vi "FA25_FW_pendulum_L3_4_0.vi"() -> ()   [LabVIEW 2024]
uses:
  <vilib>/Analysis/3filter.llb/Filter Passband Type.ctl
  SADI_Pendulum_lib/pendulumApp.lvlib
  <vilib>/ptbypt/NI_PtbyPt.lvlib
  <vilib>/Analysis/NI_AALBase.lvlib
panel:
  in  "Tab Control":T1(tab)=enum."Plant and Controller"
  out "Firmware Version":sgl=1.002
  out "Software Version":dbl=1.104 format="%_6g"
  out "Number of SADI":i32=1
  out "reset":i32
  out "SADI Connect":i32
  out "P query":i32
  out "P start":i32
  in  "Desired DAQ Loop \nTime (ms)":dbl=0.2
  out "Actual DAQ Loop \nTime (ms)":dbl=0.20860000000084256 format="%#_7g"
  out "Elapsed \nTime (s) daq loop":dbl=15.046546899999953
  out "Txlat_ms":dbl=1.778
  out "min Txlat":dbl=0.682 format="%0.6f"
  out "max TXlat":dbl=4.932 format="%0.6f"
  out "std dev TXlat":dbl=0.7050052541669608 format="%0.6f"
  out "mean  TXlat":dbl=1.2022235999999924 format="%0.6f"
  out "Tx latency, ms":T2(graph)={"X Values"=[0.70325, 0.74575, 0.7882500000000001, 0.8307500000000001, 0.8732500000000001, 0.9157500000000001, 0.95825, 1.00075, 1.04325, 1.0857500000000002, 1.1282500000000002, 1.1707500000000002, 1.2132500000000002, 1.2557500000000001, 1.2982500000000001, 1.34075, 1.38325, 1.42575, 1.46825, 1.51075, 1.55325, 1.59575, 1.63825, 1.68075, 1.72325, 1.76575, 1.8082500000000004, 1.8507500000000003, 1.8932500000000003, 1.9357500000000003, 1.9782500000000003, 2.02075, 2.06325, 2.10575, 2.14825, 2.19075, 2.23325, 2.27575, 2.31825, 2.36075, 2.40325, 2.44575, 2.48825, 2.53075, 2.57325, 2.61575, 2.65825, 2.7007499999999998, 2.7432499999999997, 2.7857499999999997, 2.8282499999999997, 2.8707499999999997, 2.9132499999999997, 2.95575, 2.99825, 3.04075, 3.08325, 3.12575, 3.16825, 3.21075, 3.25325, 3.29575, 3.33825, 3.38075, 3.42325, 3.46575, 3.50825, 3.55075, 3.59325, 3.63575, 3.67825, 3.72075, 3.7632499999999998, 3.8057499999999997, 3.84825, 3.89075, 3.93325, 3.97575, 4.01825, 4.0607500000000005, 4.10325, 4.1457500000000005, 4.18825, 4.2307500000000005, 4.27325, 4.31575, 4.35825, 4.40075, 4.44325, 4.48575, 4.52825, 4.57075, 4.61325, 4.65575, 4.698250000000001, 4.74075, 4.783250000000001, 4.82575, 4.868250000000001, 4.91075], "Histogram: h(x)"=[155, 338, 552, 840, 858, 795, 153, 0, 0, 0, 0, 0, 0, 0, 0, 0, 0, 0, 0, 0, 0, 0, 0, 5, 49, 156, 220, 199, 196, 149, 0, 0, 0, 0, 0, 0, 0, 0, 0, 0, 0, 0, 0, 0, 0, 0, 0, 17, 26, 34, 37, 44, 58, 6, 0, 0, 0, 0, 0, 0, 0, 0, 0, 0, 0, 0, 0, 0, 0, 0, 0, 5, 5, 19, 5, 41, 7, 0, 0, 0, 0, 0, 0, 0, 0, 0, 0, 0, 0, 0, 0, 0, 0, 0, 0, 4, 0, 3, 0, 24]}
  out "ENC VEL":dbl=0.5175486320891765
  out "Pend Rot Error":dbl
  out "Pend Rot Filt":dbl=nan format="%0.2f"
  out "Pendulum velocity":dbl=3.5305560095629e-285
  out "Platen velocity":dbl=0.01738392532814515
  out "Command":dbl=-14.479572053947942
  out "desired\nposition":dbl=-14.790379679306856
  out "Platen Rot Error":dbl format="%0.2f"
  in  "Frequency":dbl=0.5
  in  "Amplitude":dbl=100.0
  in  "Turn On Command":dbl=40.0
  in  "Stop":bool=TRUE
  in  "Desired Loop \nTime (ms)":dbl=1.0
  out "Actual Loop Time (ms)":dbl=1.0000979999995252
  out "Elapsed Time (s)":dbl=15.048252700000035
  out "Segments Saved":u32
  in  "Save Data?":bool
  out "ENC POS":i32=-761
  out "Pendulum ENC":i32
  in  "Sine/Square":bool=TRUE
  in  "Enable Motor":bool=TRUE
  in  "Output Units":enum16{"Degrees", "Radians"}(ring)
  in  "Couts/rev":dbl=3704.0
  in  "Zero":bool
  out "Platen Rotation":dbl=-73.96328293736501
  out "Command Graph":T3(graph)={"Desired Rotation/Command"=-14.479572053947942, -14.479572053947942, 0.0, 0.0}
  out "Desired vs Actual Platen Angle Graph":cluster{"sine wave":dbl, "Filtered x":dbl}(graph)={"sine wave"=-14.479572053947942, "Filtered x"=-73.96328293736501}
  out "Pendulum Rotation Graph":cluster{dbl, dbl}(graph)={nan, 0.0}
  in  "n-int":i32=100
  in  "n-diff":i32=5
  in  "Sampling freq: fs":dbl=1000.0
  in  "Cutoff freq: fl":dbl=10.0 format="%0.3f"
  in  "initialize":bool
  out "PendEncValMax":u16=3687
  out "PendEncValMin":u16=3178
  in  "Pendulum Zero":bool
  out "Pend Rotation":dbl=1440.0 format="%0.2f"
  out "Read Call Error Out":u16(ring)=32768 items=["SADI_RESET (FT_OK)"=0, "FT_INVALID_HANDLE"=1, "FT_DEVICE_NOT_FOUND"=2, "FT_DEVICE_NOT_OPENED"=3, "FT_IO_ERROR"=4, "FT_INSUFFICIENT_RESOURCES"=5, "FT_OTHER_ERROR"=18, "FT_NOT_SUPPORTED"=17, "DATA_RECEIVED"=32768, "NO_DATA_AVAIL"=32769, "NO_SADI"=32770]
  out "SADI State":T4(ring)=enum."Close"
  # "Platen Rotation & Velocity"
  # "Signal Generator"
  # "Butterworth Filter Settings"
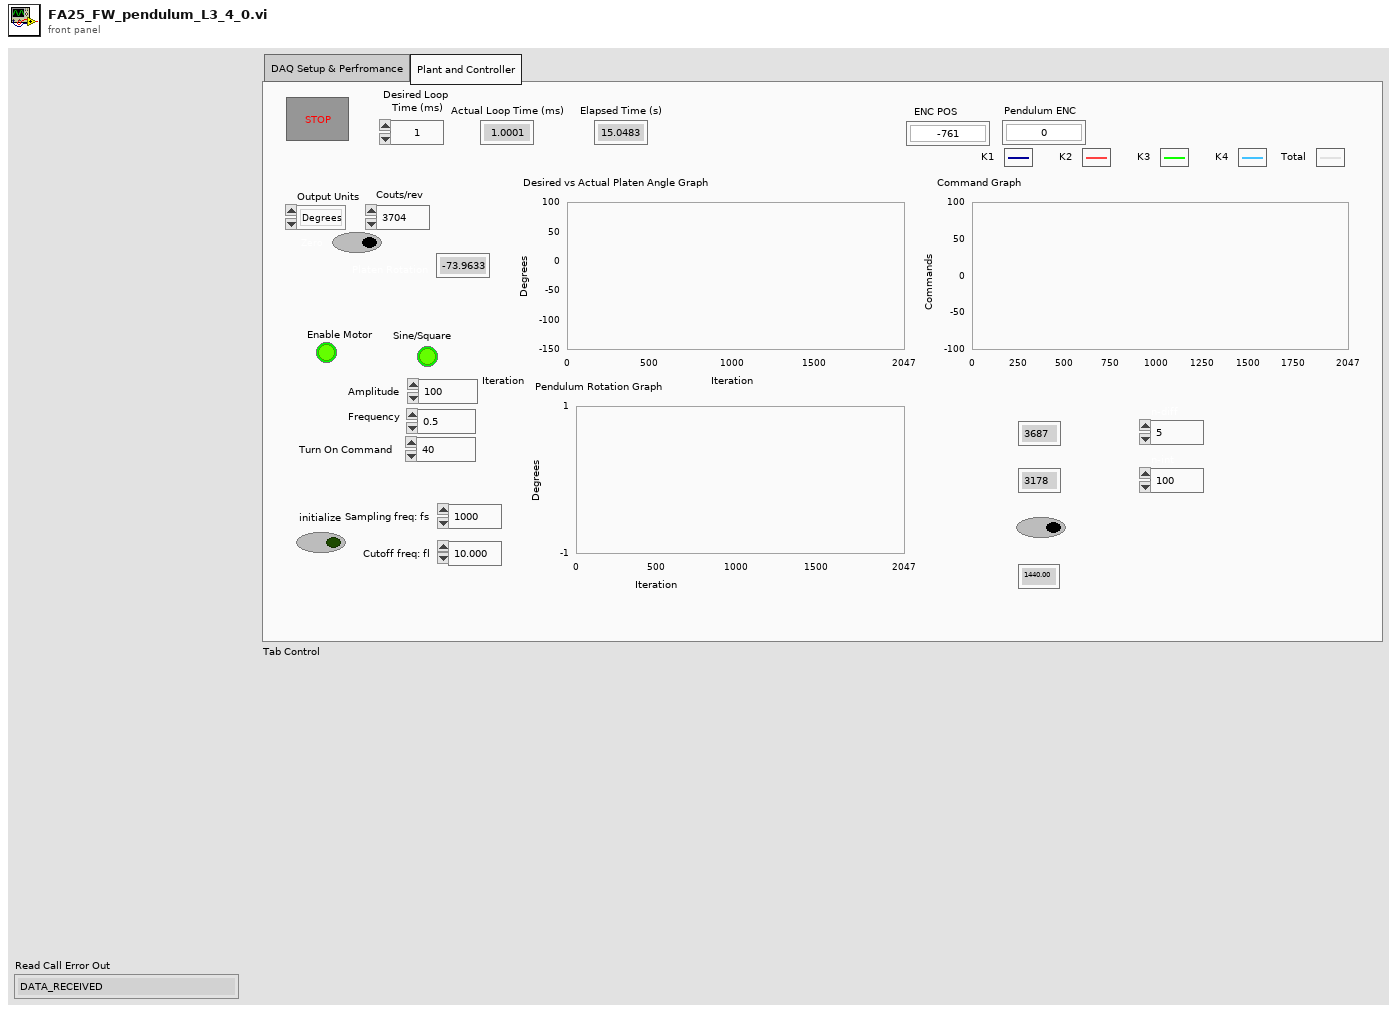
[diagram p1: front panel]
types:
  T1 = enum32{"DAQ Setup & Perfromance", "Plant and Controller"}
  T2 = cluster{"X Values":dbl[], "Histogram: h(x)":i32[]}
  T3 = cluster{"Desired Rotation/Command":dbl, dbl, dbl, dbl}
  T4 = enum32{"SADI_check", "Connect_boot", "Check_SW_FW", "Pend_Start", "Run", "Stop", "Store", "Close"}
  T5 = typedef "NI_AALBase.lvlib/Filter Passband Type.ctl" = enum32{"Lowpass", "Highpass", "Bandpass", "Bandstop"}
  T6 = cluster{"desired\nposition":dbl, "Platen Rotation":dbl}
  T7 = cluster{"desired\nposition":dbl, "Command":dbl, dbl, dbl}
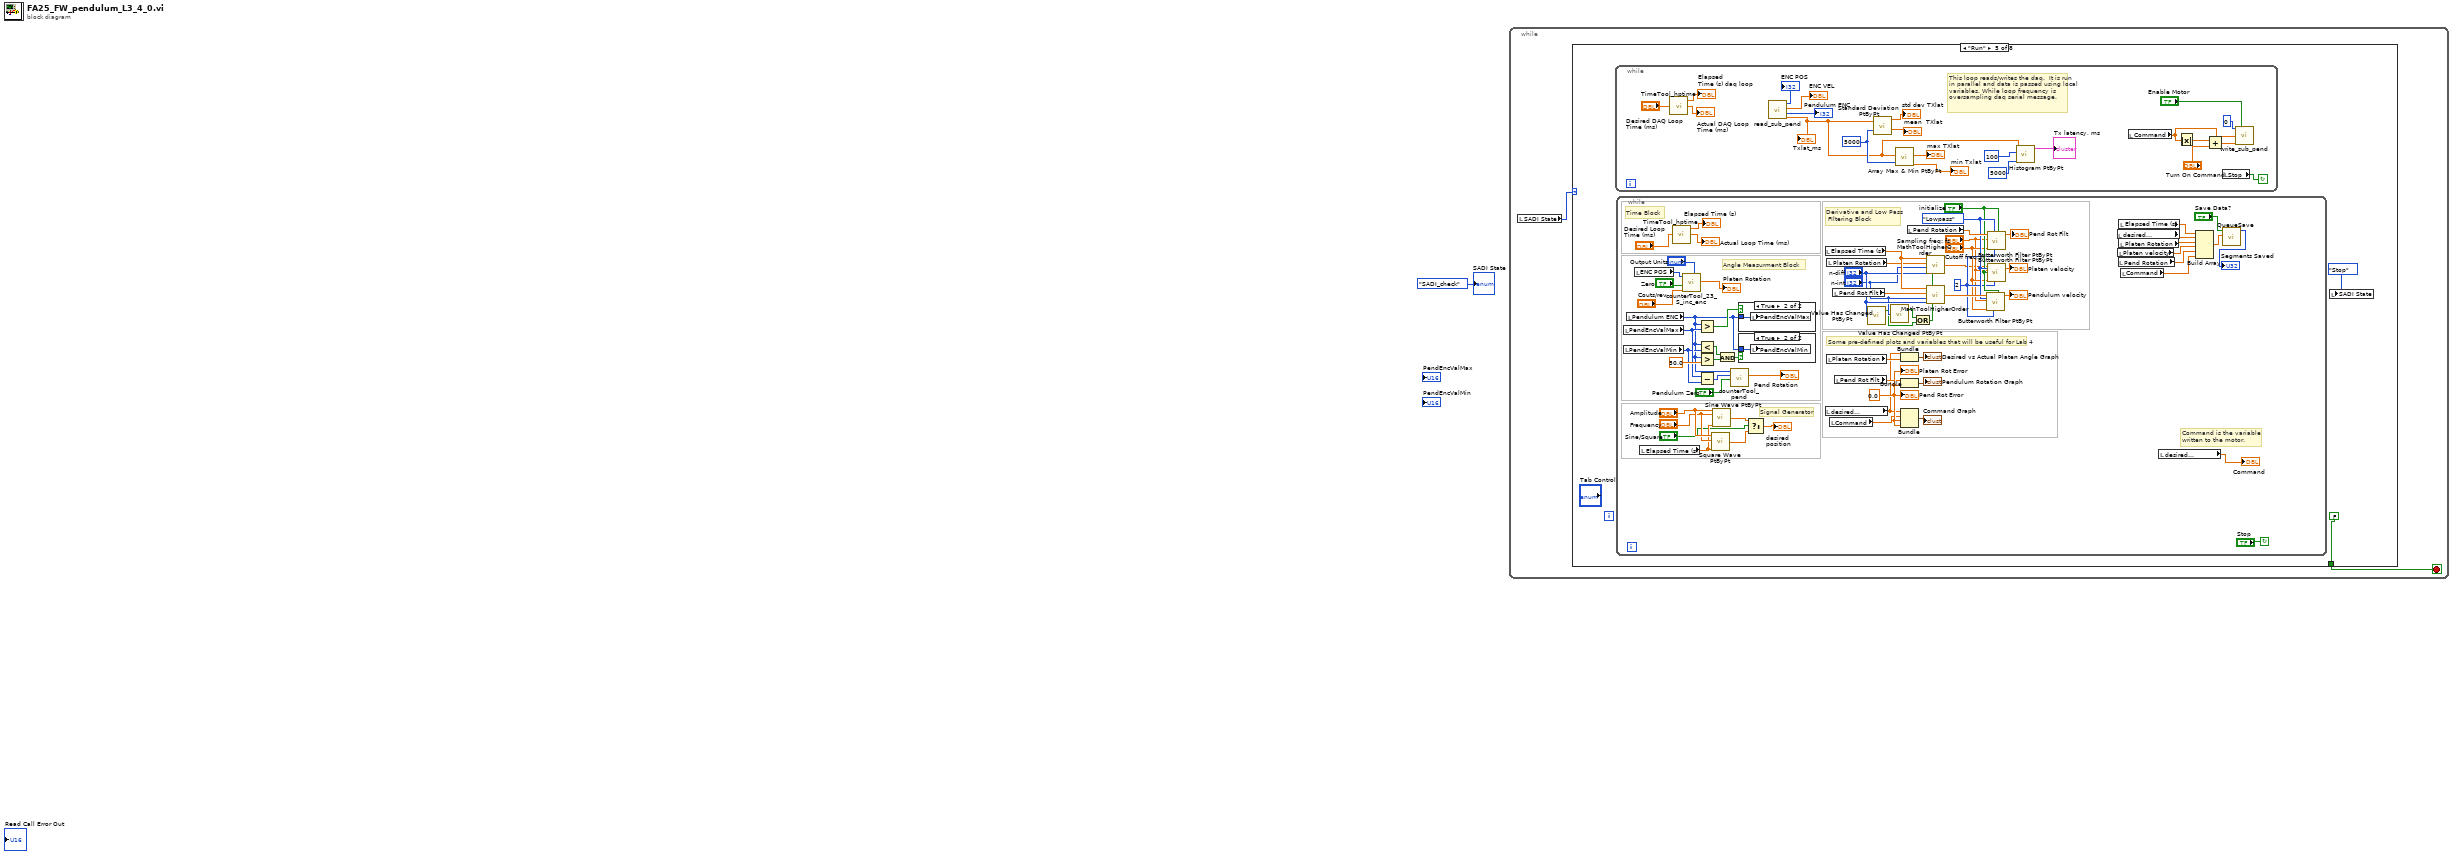
[diagram p0: block diagram]
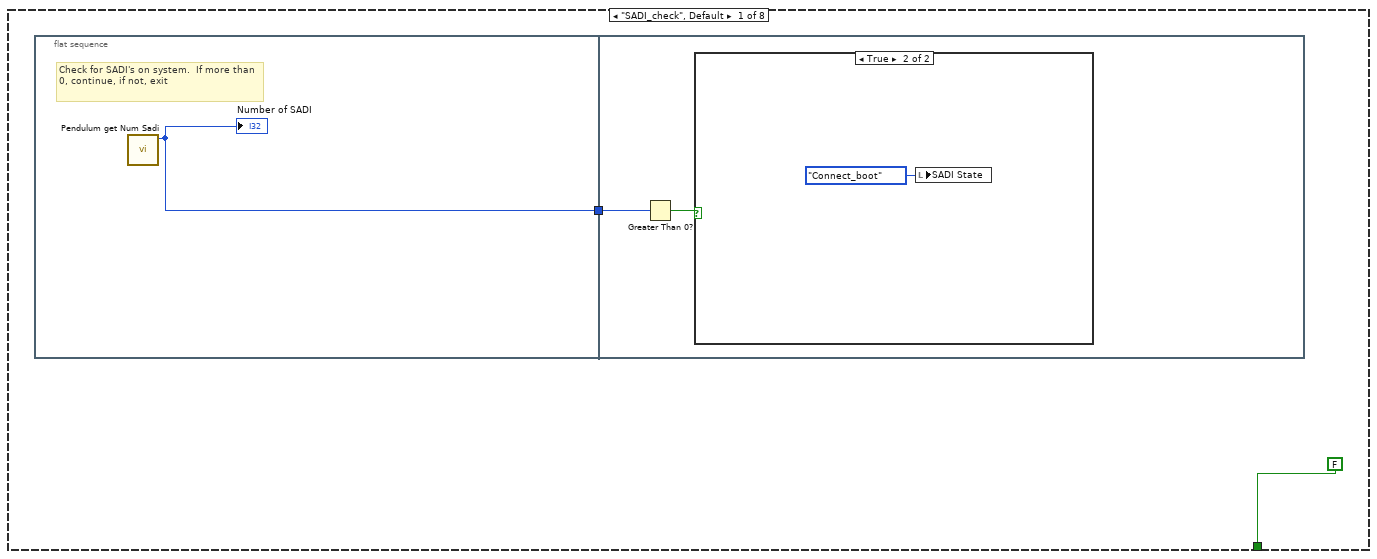
[diagram p2: hidden frame]
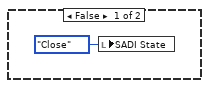
[diagram p3: hidden frame]
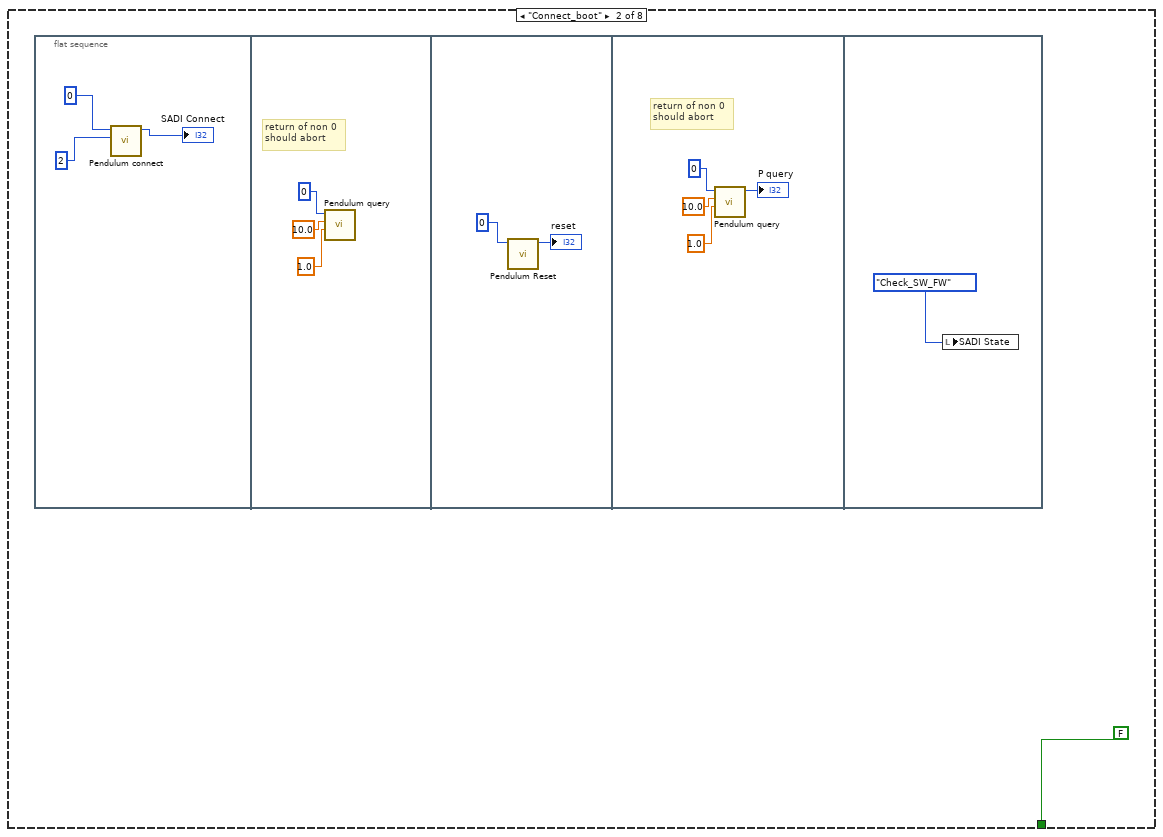
[diagram p4: hidden frame]
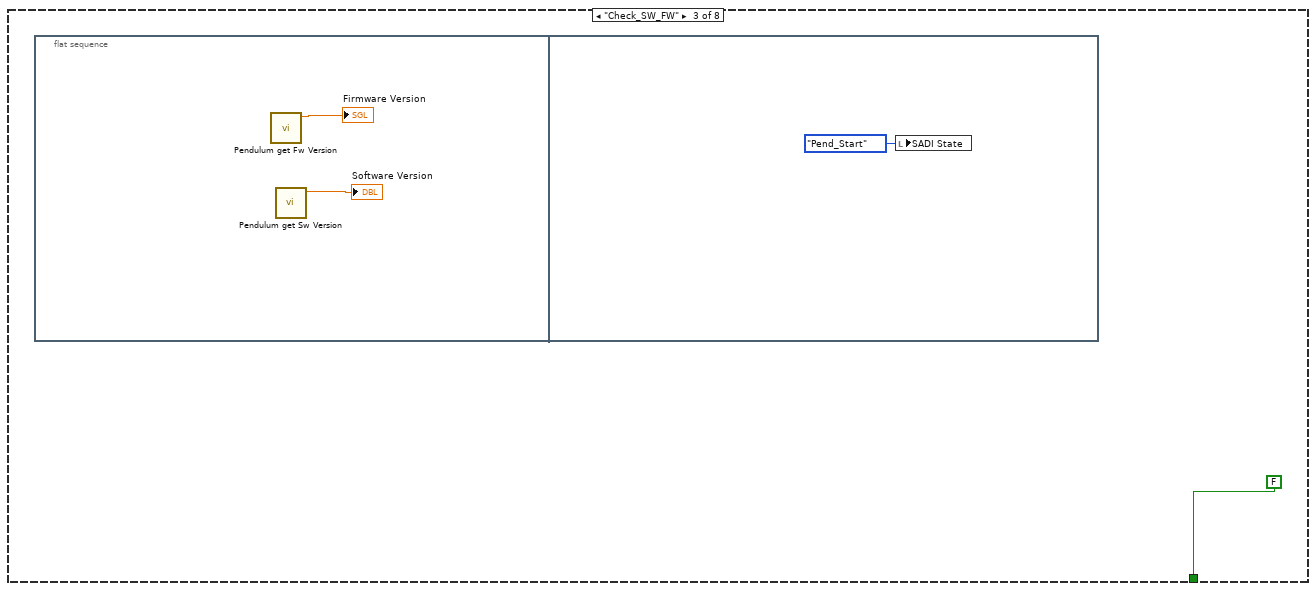
[diagram p5: hidden frame]
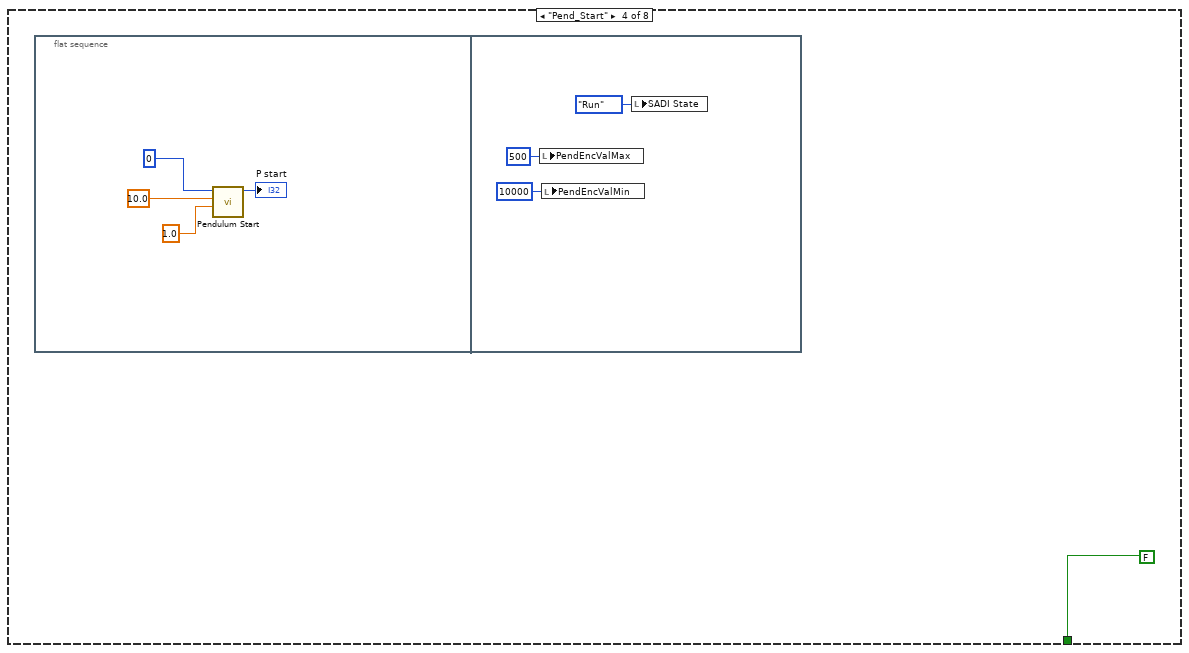
[diagram p6: hidden frame]
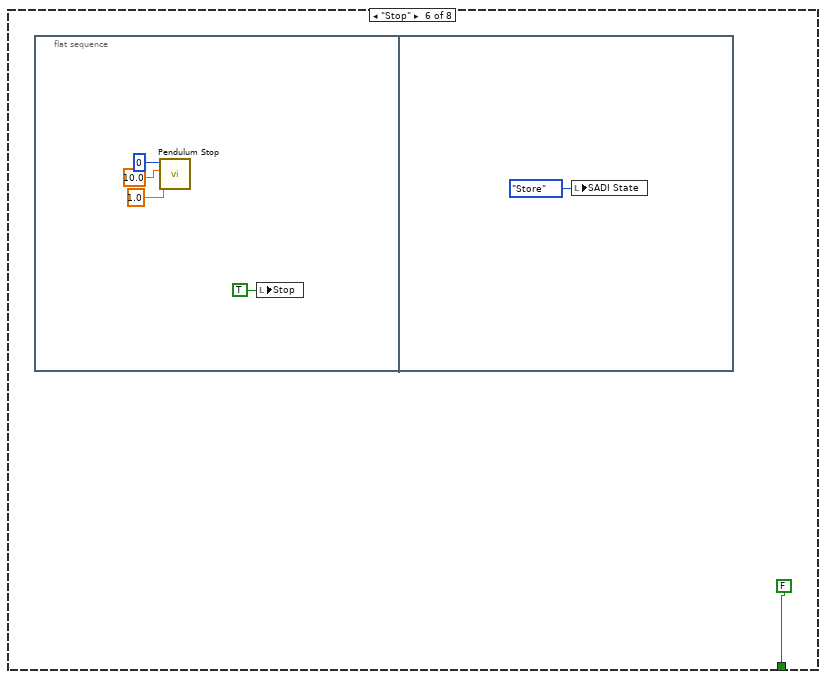
[diagram p9: hidden frame]
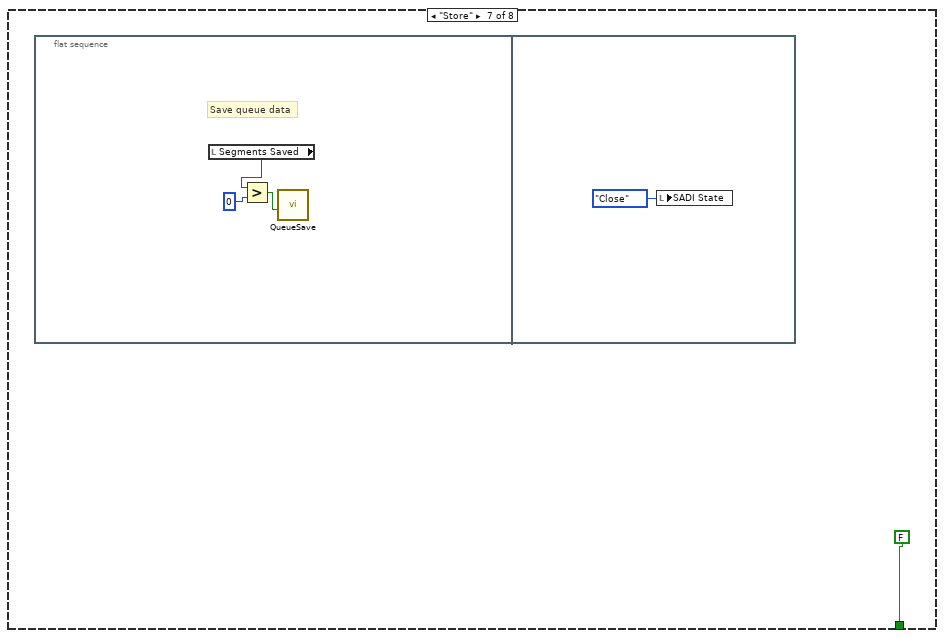
[diagram p10: hidden frame]
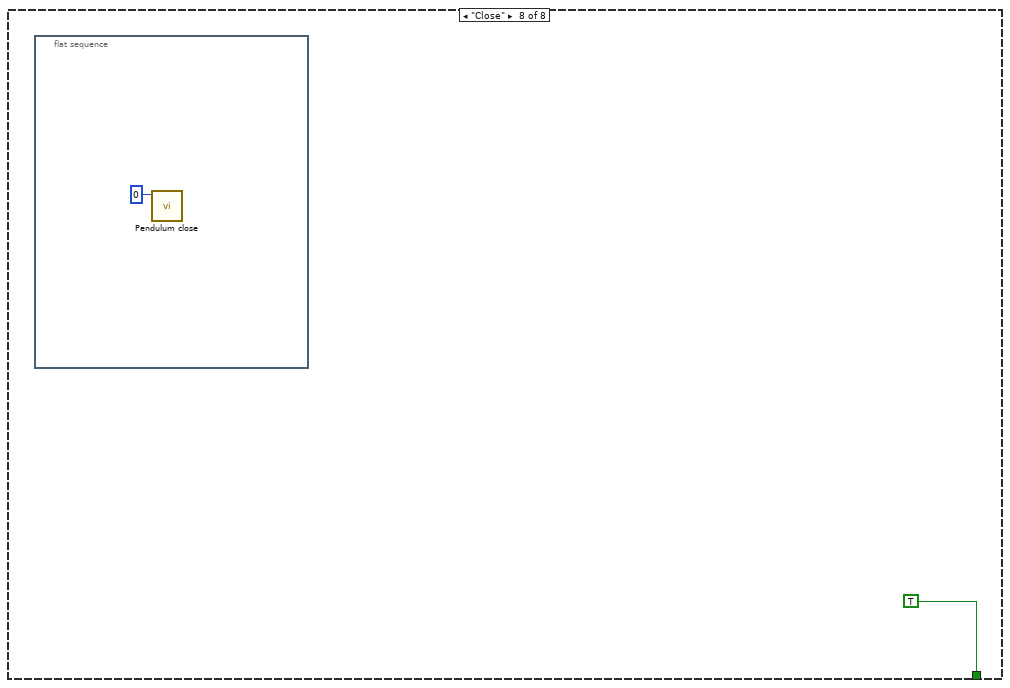
[diagram p11: hidden frame]
diagram:
  n1 = while {
    stop <- w2 stop-if-true
    n2 = local read "SADI State"() -> (w3:T4)
    n3 = case shown="\"Run\"" w3 {
      tunnel: [FALSE FALSE FALSE FALSE FALSE FALSE FALSE TRUE] -> w2
      frame "SADI_check", Default {
        n4 = flat-sequence {
          tunnel: [w6] -> w5
          tunnel: w5 -> [w7]
          frame #0 {
            # "Check for SADI's on system.  If more than 0, continue, if not, exit"
            n5 = call "Pendulum get Num Sadi.vi"() -> ("function return"=w6:i32)  [unwired: 11 in]
            "Number of SADI" <- w6
          }
          frame #1 {
            n6 = Greater Than 0?(x=w7) -> (x > 0?=w8:bool)
            n7 = case shown="True" w8 {
              frame False {
                n8 = local write "SADI State"(T4."Close" ("SADI State")) -> ()
              }
              frame True {
                n9 = local write "SADI State"(T4."Connect_boot" ("SADI State")) -> ()
              }
            }
          }
        }
      }
      frame "Connect_boot" {
        n10 = flat-sequence {
          frame #0 {
            n11 = call "Pendulum connect.vi"("latency_mS"=u8 2, "instance"=0) -> ("function return"=→"SADI Connect":i32)  [unwired: 9 in]
          }
          frame #1 {
            # "return of non 0\nshould abort"
            n12 = call "Pendulum query.vi"("timeout_sec"=1.0, "retry_ms"=10.0, "instance"=0) -> ()  [unwired: 8 in, 1 out]
          }
          frame #2 {
            n13 = call "Pendulum Reset.vi"("instance"=0) -> ("function return"=→"reset":i32)  [unwired: 10 in]
          }
          frame #3 {
            # "return of non 0\nshould abort"
            n14 = call "Pendulum query.vi"("timeout_sec"=1.0, "retry_ms"=10.0, "instance"=0) -> ("function return"=→"P query":i32)  [unwired: 8 in]
          }
          frame #4 {
            n15 = local write "SADI State"(T4."Check_SW_FW" ("SADI State")) -> ()
          }
        }
      }
      frame "Check_SW_FW" {
        n16 = flat-sequence {
          frame #0 {
            n17 = call "Pendulum get Fw Version.vi"() -> ("function return"=→"Firmware Version":dbl)  [unwired: 11 in]
            n18 = call "Pendulum get Sw Version.vi"() -> ("function return"=→"Software Version":dbl)  [unwired: 11 in]
          }
          frame #1 {
            n19 = local write "SADI State"(T4."Pend_Start" ("SADI State")) -> ()
          }
        }
      }
      frame "Pend_Start" {
        n20 = flat-sequence {
          frame #0 {
            n21 = call "Pendulum Start.vi"("timeout_sec"=1.0, "retry_mS"=10.0, "instance"=0) -> ("function return"=→"P start":i32)  [unwired: 8 in]
          }
          frame #1 {
            n22 = local write "PendEncValMax"(u16 500 ("PendEncValMax")) -> ()
            n23 = local write "PendEncValMin"(u16 10000 ("PendEncValMin")) -> ()
            n24 = local write "SADI State"(T4."Run" ("SADI State")) -> ()
          }
        }
      }
      frame "Run" {
        n25 = while {
          stop <- w40 continue-if-true
          w54 = 5000 ("sample length")
          # "This loop reads/writes the daq.  It is run in parallel and data is passed using local variables. While loop frequency is oversampling daq serial message."
          n26 = call "TimeTool_hptime.vi"("Desired Loop Time (ms)"="Desired DAQ Loop \nTime (ms)") -> ("elapsed time (s)"=→"Elapsed \nTime (s) daq loop":dbl, "dt (ms)"=→"Actual DAQ Loop \nTime (ms)":dbl)  [unwired: 1 out]
          n27 = call "read_sub_pend.vi"() -> ("Txlat_ms"=w49:dbl, "Pendulum ENC 2"=→"Pendulum ENC":i32, "ENC VEL 1"=→"ENC VEL":dbl, "ENC POS 1"=→"ENC POS":i32)  [unwired: 7 in]
          "Txlat_ms" <- w49
          n28 = call <vilib>:"Standard Deviation PtByPt.vi"("x"=w49, "sample length"=w54) -> ("standard deviation"=→"std dev TXlat":dbl, "mean"=→"mean  TXlat":dbl)  [unwired: 1 in, 1 out]
          n29 = call <vilib>:"Array Max & Min PtByPt.vi"("input data point"=w49, "sample length"=w54) -> ("max value"=→"max TXlat":dbl, "min value"=→"min Txlat":dbl)  [unwired: 1 in, 3 out]
          n30 = call <vilib>:"Histogram PtByPt.vi"("sample length"=5000, "intervals"=100, "x"=w49) -> ("Histogram Graph"=→"Tx latency, ms":T2)  [unwired: 5 in, 3 out]
          n31 = local read "Command"() -> (w39:dbl)
          n32 = Absolute Value(x=w39) -> (abs(x)=w45:dbl)
          n33 = Add(x=w45, y="Turn On Command") -> (x+y=w46:dbl)
          n34 = local read "Stop"() -> (w40:bool)
          n35 = call "write_sub_pend.vi"("instance"=0, "Enable Motor"="Enable Motor", "direction"=w39, "motorEffort"=w46) -> ()  [unwired: 12 in]
        }
        n36 = while {
          stop <- "Stop" continue-if-true
          w70 = 0.0
          w80 = 2 ("order")
          w82 = Filter_Passband_Type."Lowpass" ("filter type")
          # "Command is the variable \nwritten to the motor."
          # "Some pre-defined plots and variables that will be useful for Lab 4"
          # "Derivative and Low Pass\n FIltering Block"
          # "Angle Measurment Block"
          # "Signal Generator"
          # "Time Block"
          n37 = local read "PendEncValMax"() -> (w96:u16)
          n38 = local read "PendEncValMin"() -> (w95:u16)
          n39 = local read "Pendulum ENC"() -> (w93:i32)
          n40 = local read "ENC POS"() -> (w107:i32)
          n41 = local read "Elapsed Time (s)"() -> (w115:dbl)
          n42 = call "TimeTool_hptime.vi"("Desired Loop Time (ms)"="Desired Loop \nTime (ms)") -> ("elapsed time (s)"=→"Elapsed Time (s)":dbl, "dt (ms)"=→"Actual Loop Time (ms)":dbl)  [unwired: 1 out]
          n43 = call "counterTool_23_S_inc_enc.vi"("Counts"=w107, "Zero"="Zero", "Couts/rev"="Couts/rev", "Output Units"="Output Units") -> ("Total Angle"=→"Platen Rotation":dbl)  [unwired: 3 in, 1 out]
          n44 = Greater?(x=w93, y=w96) -> (0:w100:bool)
          n45 = Less?(x=w93, y=w95) -> (x < y?=w102:bool)
          n46 = Greater?(x=w93, y=50.0) -> (0:w101:bool)
          n47 = Subtract(x=w96, y=w95) -> (x-y=w97:u16)
          n48 = call <vilib>:"Square Wave PtByPt.vi"("amplitude"="Amplitude", "frequency"="Frequency", "time"=w115) -> ("square wave"=w112:dbl)  [unwired: 2 in]
          n49 = call <vilib>:"Sine Wave PtByPt.vi"("time"=w115, "frequency"="Frequency", "amplitude"="Amplitude") -> ("sine wave"=w113:dbl)  [unwired: 1 in]
          n50 = And(x=w102, y=w101) -> (x .and. y?=w99:bool)
          n51 = call "counterTool_pend.vi"("Counts"=w93, "Pendulum Scale"=w97, "Zero"="Pendulum Zero") -> ("Total Angle"=→"Pend Rotation":dbl)  [unwired: 4 in, 1 out]
          n52 = case shown="True" w100 {
            tunnel: w93 -> [_ w126]
            frame False {
            }
            frame True {
              n53 = local write "PendEncValMax"(w126) -> ()
            }
          }
          n54 = case shown="True" w99 {
            tunnel: w93 -> [_ w125]
            frame False {
            }
            frame True {
              n55 = local write "PendEncValMin"(w125) -> ()
            }
          }
          n56 = Select(t=w113, s="Sine/Square", f=w112) -> (s? t:f=→"desired\nposition":dbl)
          n57 = local read "Elapsed Time (s)"() -> (w91:dbl)
          n58 = local read "desired\nposition"() -> (w62:dbl)
          n59 = local read "Platen Rotation"() -> (w69:dbl)
          n60 = local read "Platen Rotation"() -> (w86:dbl)
          n61 = local read "Command"() -> (w61:dbl)
          n62 = local read "Pend Rot Filt"() -> (w85:dbl)
          n63 = local read "Pend Rot Filt"() -> (w68:dbl)
          n64 = call <vilib>:"Value Has Changed PtByPt.vi"("input data point"="n-diff") -> ("has changed"=w74:bool)  [unwired: 1 in, 1 out]
          n65 = call <vilib>:"Value Has Changed PtByPt.vi"("input data point"="n-int") -> ("has changed"=w75:bool)  [unwired: 1 in, 1 out]
          n66 = Bundle("desired\nposition"=w62, "Platen Rotation"=w69) -> (→"Desired vs Actual Platen Angle Graph":T6)  [unwired: 1 in]
          n67 = Bundle("Pend Rot Filt"=w68, w70) -> (→"Pendulum Rotation Graph":cluster{"Pend Rot Filt":dbl, dbl})  [unwired: 1 in]
          n68 = Bundle("desired\nposition"=w62, "Command"=w61, w70, w70) -> (→"Command Graph":T7)  [unwired: 1 in]
          n69 = local read "Pend Rotation"() -> (w87:dbl)
          n70 = Or(x=w75, y=w74) -> (x .or. y?=w89:bool)
          n71 = call "MathToolHigherOrder.vi"("Time"=w91, "Data"=w86, "n-int"="n-int", "Reset (F)"=w89, "n-diff"="n-diff") -> ("1st derivative"=w76:dbl)  [unwired: 1 in, 2 out]
          n72 = call "MathToolHigherOrder.vi"("Time"=w91, "Data"=w85, "n-int"="n-int", "Reset (F)"=w89, "n-diff"="n-diff") -> ("1st derivative"=w83:dbl)  [unwired: 1 in, 2 out]
          n73 = call <vilib>:"Butterworth Filter PtByPt.vi"("initialize"="initialize", "order"=w80, "filter type"=w82, "low cutoff freq: fl"="Cutoff freq: fl", "sampling freq: fs"="Sampling freq: fs", "x"=w83) -> ("Filtered x"=→"Pendulum velocity":dbl)  [unwired: 3 in, 1 out]
          n74 = call <vilib>:"Butterworth Filter PtByPt.vi"("initialize"="initialize", "order"=w80, "filter type"=w82, "low cutoff freq: fl"="Cutoff freq: fl", "sampling freq: fs"="Sampling freq: fs", "x"=w87) -> ("Filtered x"=→"Pend Rot Filt":dbl)  [unwired: 3 in, 1 out]
          n75 = call <vilib>:"Butterworth Filter PtByPt.vi"("initialize"="initialize", "order"=w80, "filter type"=w82, "low cutoff freq: fl"="Cutoff freq: fl", "sampling freq: fs"="Sampling freq: fs", "x"=w76) -> ("Filtered x"=→"Platen velocity":dbl)  [unwired: 3 in, 1 out]
          n76 = local read "desired\nposition"() -> (w104:dbl)
          n77 = local read "Platen velocity"() -> (w66:dbl)
          n78 = local read "Pend Rotation"() -> (w65:dbl)
          n79 = local read "Elapsed Time (s)"() -> (w123:dbl)
          n80 = local read "Platen Rotation"() -> (w67:dbl)
          n81 = local read "Command"() -> (w64:dbl)
          n82 = local read "desired\nposition"() -> (→"Command":dbl)
          n83 = Build Array(w123, w104, w67, w66, w65, w64) -> (w122:dbl[])
          n84 = call "QueueSave.vi"("Data In"=w122, "Save Data?"="Save Data?") -> ("Segments Saved"=→"Segments Saved":u32)  [unwired: 3 in, 2 out]
          "Platen Rot Error" <- w70
          "Pend Rot Error" <- w70
        }
        n85 = local write "SADI State"(T4."Stop" ("SADI State")) -> ()
      }
      frame "Stop" {
        n86 = flat-sequence {
          frame #0 {
            n87 = call "Pendulum Stop.vi"("timeout_sec"=1.0, "retry_mS"=10.0, "instance"=0) -> ()  [unwired: 8 in, 1 out]
            n88 = local write "Stop"(TRUE ("Stop")) -> ()
          }
          frame #1 {
            n89 = local write "SADI State"(T4."Store" ("SADI State")) -> ()
          }
        }
      }
      frame "Store" {
        n90 = flat-sequence {
          frame #0 {
            # "Save queue data"
            n91 = local read "Segments Saved"() -> (w136:u32)
            n92 = Greater?(x=w136, y=u32 0) -> (0:w135:bool)
            n93 = call "QueueSave.vi"("Write To Spreadsheet"=w135) -> ()  [unwired: 4 in, 3 out]
          }
          frame #1 {
            n94 = local write "SADI State"(T4."Close" ("SADI State")) -> ()
          }
        }
      }
      frame "Close" {
        n95 = flat-sequence {
          frame #0 {
            n96 = call "Pendulum close.vi"("instance"=0) -> ()  [unwired: 10 in, 1 out]
          }
        }
      }
    }
  }
  "SADI State" <- T4."SADI_check" ("SADI State")
